vi "PRIME Telescope Focus Move.vi"(8 "error in (no error)":errorcluster, 10 "focus pos":dbl, 11 "connection ID":refnum<k5>) -> (0 "error out":errorcluster)   [LabVIEW 2021, in "PRIME Telescope.lvclass"]
uses:
  PRIME Telescope.lvclass
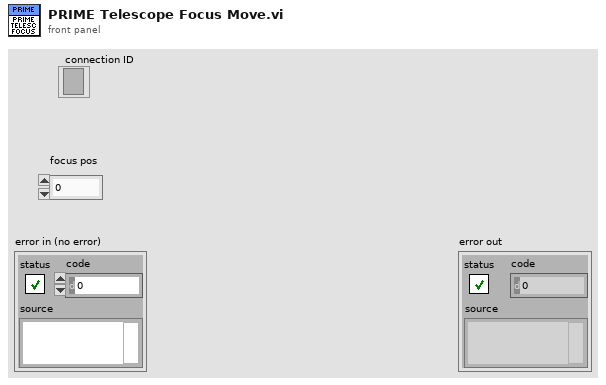
[diagram p1: front panel]
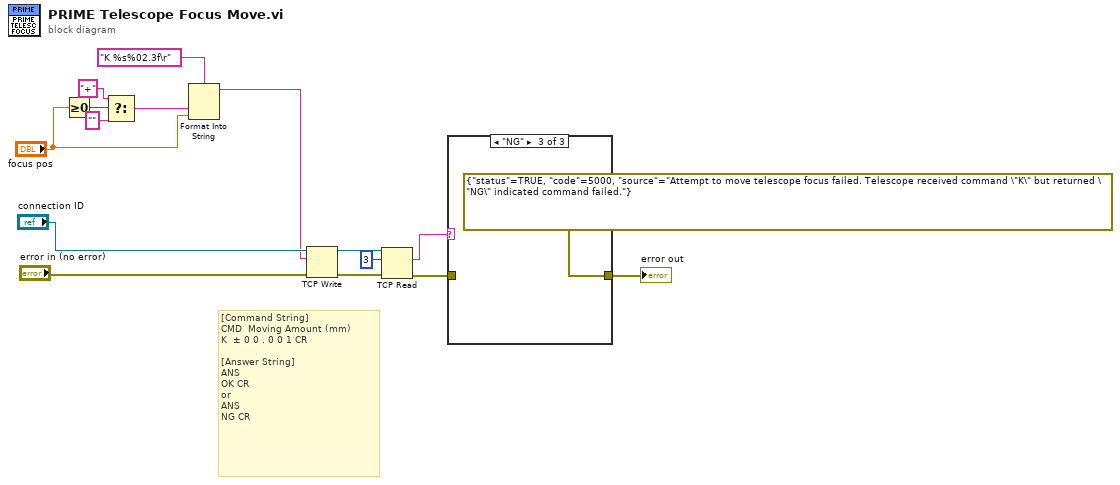
[diagram p0: block diagram]
diagram:
  # "[Command String]\nCMD\t\tMoving Amount (mm)\t\nK\t\t±\t0\t0\t.\t0\t0\t1\tCR\n\n[Answer String]\nANS\t\nOK\tCR\nor\nANS\t\nNG\tCR"
  n1 = Greater Or Equal To 0?(x="focus pos") -> (x >= 0?=w10:bool)
  n2 = Select(t="+", s=w10, f="") -> (s? t:f=w6:string)
  n3 = Format Into String(format string="K %s%02.3f\r", w6, "focus pos") -> (resulting string=w4:string)  [unwired: 2 in, 1 out]
  n4 = TCP Write(connection ID="connection ID", data in=w4, error in (no error)="error in (no error)") -> (connection ID out=w14:refnum<k5>, error out=w15:errorcluster)  [unwired: 1 in, 1 out]
  n5 = TCP Read(connection ID=w14, bytes to read=3, error in (no error)=w15) -> (data out=w2:string, error out=w3:errorcluster)  [unwired: 2 in, 1 out]
  n6 = case shown="\"NG\"" w2 {
    tunnel: w3 -> [w16 w17 _]
    tunnel: [w16 w17 errorcluster {"status"=TRUE, "code"=5000, "source"="Attempt to move telescope focus failed. Telescope received command \"K\" but returned \"NG\" indicated command failed."} ("error out")] -> w1
    frame "False", Default {
    }
    frame "OK" {
    }
    frame "NG" {
    }
  }
  "error out" <- w1
